vi "debug_fg.vi"(7 "action":T1, 8 "error in (no error)":errorcluster, 11 "data":string) -> (0 "error out":errorcluster, 3 "debug":string)   [LabVIEW 2017, in "rethinkdb.lvlib"]
uses:
  rethinkdb.lvlib
  debug_action.ctl
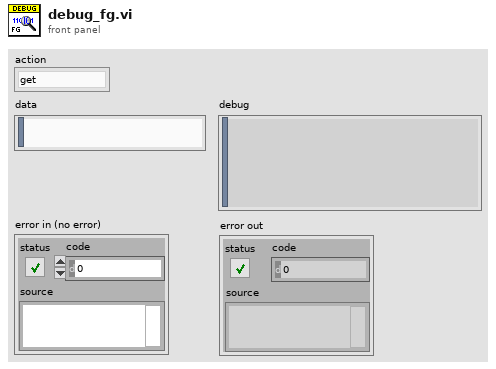
[diagram p1: front panel]
types:
  T1 = typedef "rethinkdb.lvlib/debug_action.ctl" = enum8{"get", "set_query", "set_response", "clear"}
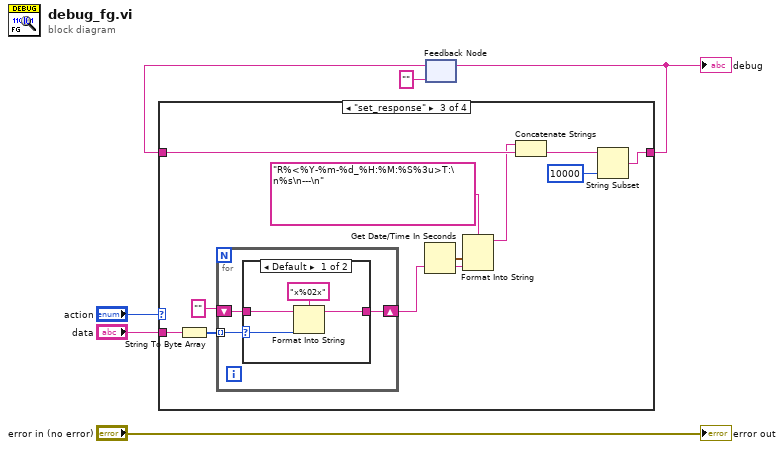
[diagram p0: block diagram]
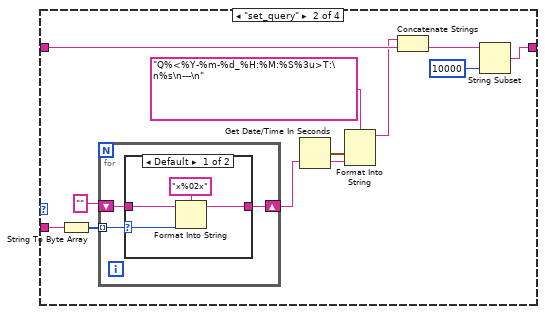
[diagram p3: hidden frame]
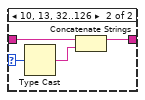
[diagram p4: hidden frame]
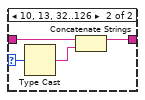
[diagram p5: hidden frame]
diagram:
  n1 = feedback #1("") -> (w3:string)
  n2 = case shown="\"set_response\"" "action" {
    tunnel: w3 -> [w7 w18 w40 _]
    tunnel: [w7 w13 w35 _] -> w2
    tunnel: "data" -> [_ w10 w32 _]
    frame "get" {
    }
    frame "set_query" {
      n3 = String To Byte Array(string=w10) -> (unsigned byte array=w12:u8[])
      n4 = for {
        tunnel: w12 -> [w20] mode=indexing
        shift-right: [w19] -> w8
        shift-left: "" -> [w21]
        n5 = case shown="Default" w20 {
          selector: w20 -> [w23 w28]
          tunnel: w21 -> [w25 w29]
          tunnel: [w24 w27] -> w19
          frame Default {
            n6 = Format Into String(format string="x%02x", initial string=w25, w23) -> (resulting string=w24:string)  [unwired: 1 in, 1 out]
          }
          frame 10, 13, 32..126 {
            n7 = Type Cast(x=w28) -> (*(type *) &x=w26:string)  [unwired: 1 in]
            n8 = Concatenate Strings(w29, w26) -> (w27:string)
          }
        }
      }
      n9 = Get Date/Time In Seconds() -> (seconds since 1Jan1904=w9:timestamp)
      n10 = Format Into String(format string="Q%<%Y-%m-%d_%H:%M:%S%3u>T:\n%s\n---\n", w9, w8) -> (resulting string=w17:string)  [unwired: 2 in, 1 out]
      n11 = Concatenate Strings(w17, w18) -> (w14:string)
      n12 = String Subset(string=w14, length (rest)=10000 ("length (rest)")) -> (substring=w13:string)  [unwired: 1 in]
    }
    frame "set_response" {
      n13 = String To Byte Array(string=w32) -> (unsigned byte array=w34:u8[])
      n14 = for {
        tunnel: w34 -> [w42] mode=indexing
        shift-right: [w41] -> w30
        shift-left: "" -> [w43]
        n15 = case shown="Default" w42 {
          selector: w42 -> [w45 w50]
          tunnel: w43 -> [w47 w51]
          tunnel: [w46 w49] -> w41
          frame Default {
            n16 = Format Into String(format string="x%02x", initial string=w47, w45) -> (resulting string=w46:string)  [unwired: 1 in, 1 out]
          }
          frame 10, 13, 32..126 {
            n17 = Type Cast(x=w50) -> (*(type *) &x=w48:string)  [unwired: 1 in]
            n18 = Concatenate Strings(w51, w48) -> (w49:string)
          }
        }
      }
      n19 = Get Date/Time In Seconds() -> (seconds since 1Jan1904=w31:timestamp)
      n20 = Format Into String(format string="R%<%Y-%m-%d_%H:%M:%S%3u>T:\n%s\n---\n", w31, w30) -> (resulting string=w39:string)  [unwired: 2 in, 1 out]
      n21 = Concatenate Strings(w39, w40) -> (w36:string)
      n22 = String Subset(string=w36, length (rest)=10000 ("length (rest)")) -> (substring=w35:string)  [unwired: 1 in]
    }
    frame "clear" {
    }
  }
  "debug" <- w2
  n23 = feedback-in #1(w2) -> ()
  "error out" <- "error in (no error)"
